vi "Input User Settings.vi"(9 "System Mode":enum16{"Off", "Cool", "Auto", "Heat"}(ring), 10 "Interval":T1, 11 "System Status Displays in":T2) -> (3 "System Status Displays out":T2)   [LabVIEW 2026]
uses:
  controls/System Status Displays.ctl
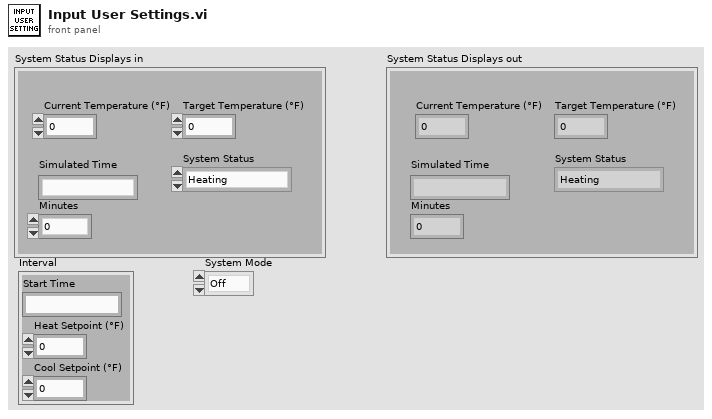
[diagram p1: front panel]
types:
  T1 = cluster{"Start Time":string, "Heat Setpoint (°F)":dbl, "Cool Setpoint (°F)":dbl}
  T2 = typedef "System Status Displays.ctl" = cluster{"Current Temperature (°F)":dbl, "Target Temperature (°F)":dbl, "System Status":enum16{"Heating", "Cooling", "Idle"}, "Simulated Time":string, "Minutes":i16}
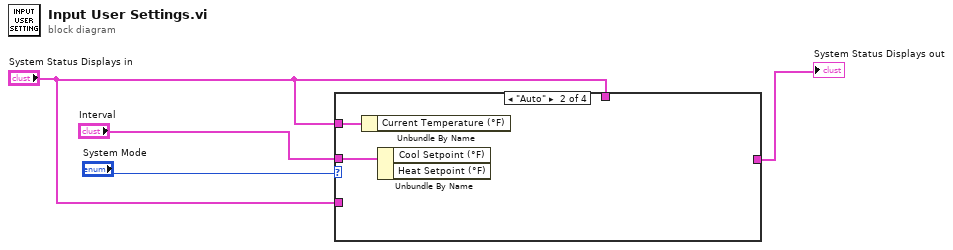
[diagram p0: block diagram]
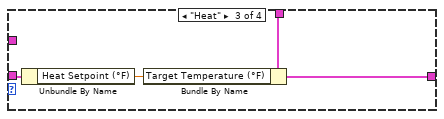
[diagram p3: hidden frame]
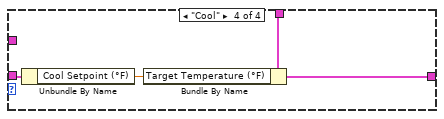
[diagram p4: hidden frame]
diagram:
  n1 = case shown="\"Auto\"" "System Mode" {
    tunnel: "System Status Displays in" -> [_ _ w11 w15]
    tunnel: "Interval" -> [_ w7 w10 w14]
    tunnel: [w5 _ w9 w13] -> w3
    tunnel: "System Status Displays in" -> [w5 _ _ _]
    tunnel: "System Status Displays in" -> [_ w6 _ _]
    frame "Off", Default {
    }
    frame "Auto" {
      n2 = Unbundle By Name(w6) -> ()  [unwired: 1 out]
      n3 = Unbundle By Name(w7) -> ()  [unwired: 2 out]
    }
    frame "Heat" {
      n4 = Unbundle By Name(w10) -> ("Heat Setpoint (°F)"=w8:dbl)
      n5 = Bundle By Name(cluster=w11, "Target Temperature (°F)"=w8) -> (w9:T2)
    }
    frame "Cool" {
      n6 = Unbundle By Name(w14) -> ("Cool Setpoint (°F)"=w12:dbl)
      n7 = Bundle By Name(cluster=w15, "Target Temperature (°F)"=w12) -> (w13:T2)
    }
  }
  "System Status Displays out" <- w3
